vi "InitShower.vi"(8 "error in (no error)":errorcluster caption="错误输入（无错误）", 10 "DevInfo":refnum<vi>, 11 "顯示框":refnum<vi>) -> (0 "error out":errorcluster caption="错误输出")   [LabVIEW 2012]
uses:
  <vilib>/Utility/miscctls.llb/LVRowAndColumnTypeDef.ctl
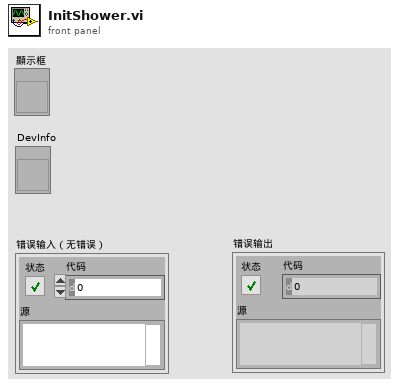
[diagram p1: front panel]
types:
  T1 = typedef "LVRowAndColumnTypeDef.ctl" = cluster{"Row":i32, "Column":i32}
  T2 = typedef "DevControl.lvclass/DevState.ctl" = enum16{"Shutdown", "PASS", "FAIL", "Idle", "Noresponse"}
  T3 = cluster{"Addr":u8, "name":string, "State":T2, "Retry":i32}[]
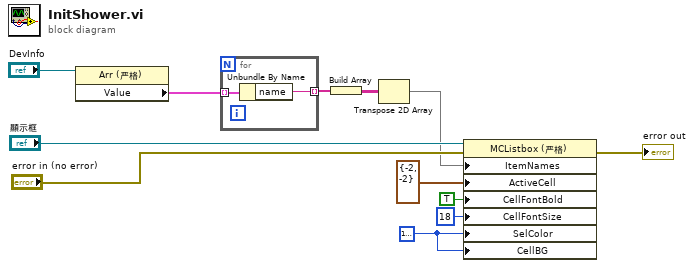
[diagram p0: block diagram]
diagram:
  w2 = u32 16777216
  n1 = property class="Arr (严格)"(reference="DevInfo") -> ("Value"=w12:T3)  [unwired: 1 in, 2 out]
  n2 = for {
    tunnel: w12 -> [w14] mode=indexing
    tunnel: [w13] -> w10 mode=indexing
    n3 = Unbundle By Name(w14) -> ("name"=w13:string)
  }
  n4 = Build Array(w10) -> (w4:string[][])
  n5 = Transpose 2D Array(2D array=w4) -> (transposed array=w3:string[][])
  n6 = property class="MCListbox (严格)"(reference="顯示框", error in="error in (no error)", "ItemNames"=w3, "ActiveCell"=T1 {"Row"=-2, "Column"=-2} ("活动单元格:活动单元格"), "CellFontBold"=TRUE ("活动单元格:单元格字体:粗体"), "CellFontSize"=u32 18 ("活动单元格:单元格字体:字号"), "SelColor"=w2, "CellBG"=w2) -> (error out=→"error out":errorcluster)  [unwired: 1 out]
